vi "发送UIErrorHandler.vi"(7 "Message Priority (Normal)":T1=enum."Normal" caption="消息优先级（标准）", 8 "error in (no error)":errorcluster caption="错误输入（无错误）", 10 "error in":errorcluster caption="错误输入（无错误）", 11 "Message Enqueuer":refnum<class "Message Enqueuer.lvclass"> caption="消息待入队列") -> (0 "error out":errorcluster caption="错误输出", 3 "Message Enqueuer out":refnum<class "Message Enqueuer.lvclass"> caption="消息待入队列输出")   [LabVIEW 2019, in "ErrorHanlder.lvlib" / "UIErrorHandler消息.lvclass"]
doc: "本VI将消息发送至操作者。"
uses:
  <vilib>/ActorFramework/Message Enqueuer/Message Enqueuer.lvclass
  <vilib>/ActorFramework/Message Enqueuer/Message Priority.ctl
  C:/Program Files (x86)/National Instruments/LabVIEW 2019/vi.lib/ActorFramework/Message/Message.lvclass
  <vilib>/ActorFramework/Message Enqueuer/Message Enqueuer.lvclass/Message Enqueuer.ctl
  <vilib>/ActorFramework/Message Priority Queue/Priority Enqueue.vi
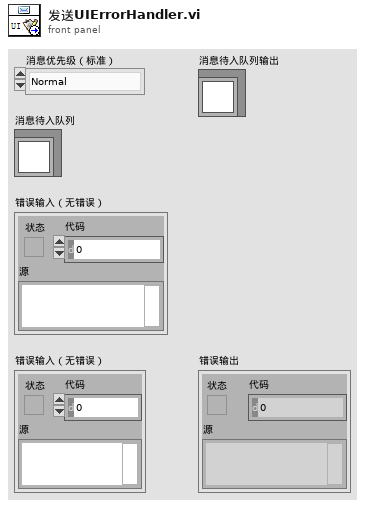
[diagram p1: front panel]
types:
  T1 = typedef "Actor Framework.lvlib/Message Enqueuer.lvclass/Message Priority.ctl" = enum16{"Low", "Normal", "High"}
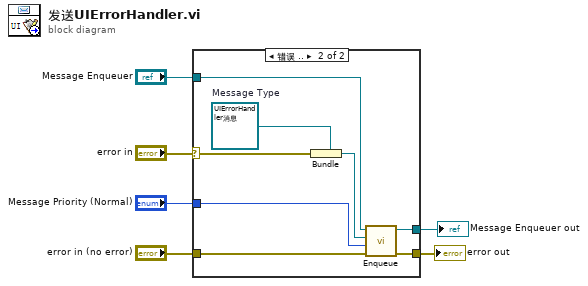
[diagram p0: block diagram]
diagram:
  n1 = case shown="错误 .." "error in" {
    selector: "error in" -> [_ w11]
    tunnel: "Message Enqueuer" -> [w8 w16]
    tunnel: "error in (no error)" -> [w7 w15]
    tunnel: [w7 w14] -> w5
    tunnel: "Message Priority (Normal)" -> [_ w13]
    tunnel: [w8 w12] -> w3
    frame No Error {
    }
    frame Error {
      w9 = refnum<class "UIErrorHandler消息.lvclass"> refnum  # Message Type
      n2 = Bundle(cluster=w9, w11) -> (w10:refnum<class "UIErrorHandler消息.lvclass">)
      n3 = call <vilib>:"Enqueue.vi"("error in (no error)"=w15, "Message Priority (Normal)"=w13, "Message"=w10, "Message Enqueuer in"=w16) -> ("error out"=w14:errorcluster, "Message Enqueuer out"=w12:refnum<class "Message Enqueuer.lvclass">)  [unwired: 6 in]
    }
  }
  "error out" <- w5
  "Message Enqueuer out" <- w3
